vi "Autonomous Independent.vi"   [LabVIEW 2017]
doc: "This VI is called when autonomous begins, and will automatically be terminated when autonomous ends. You can carry out timed or sensor driven robot movement independently without needing to return to the caller."
uses:
  <vilib>/Rock Robotics/WPI/Utilities/WPI_GetSetVariantRefNum.vi
  <vilib>/Rock Robotics/Network Tables/NT Read String.vi
  <vilib>/Rock Robotics/Network Tables/NT Write Numeric Array.vi
  <vilib>/Rock Robotics/WPI/RobotDrive/WPI_RobotDriveArcadeDrive_Standard(NoSaturation).vi
panel:
  # "Be sure to right-click and choose Data Operations>>Make Current Value default if you want to save the array values with the VI"
types:
  T1 = typedef "WPI_JoystickDevRef.ctl" = cluster{"Device":T2}
  T2 = typedef "WPI_JoystickDeviceEnum.ctl" = enum16{"USB 0", "USB 1", "USB 2", "USB 3", "USB 4", "USB 5"}
  T3 = typedef "WPI_RobotDriveDevRef.ctl" = cluster{"DevStatus":errorcluster, "Motors[]":T4[], "Square Inputs":bool, "Max Output":dbl}
  T4 = typedef "WPI_MotorControlDeviceRef.ctl" = cluster{"DeviceStatus":errorcluster, "Type":T5, "PWM":cluster{"PWM Channel":T6, "DeadBand":T7}, "CAN":cluster{"Device Number":u8, "SetOutput VI Ref":variant, "GetOutput VI Ref":variant, "Enable VI Ref":variant, "Disable VI Ref":variant, "Data":variant}, "Invert":bool, "DIO PWM":cluster{"PWM \"Enable\" Channel":T6, "DIOChannel":T8, "PWM Rate":dbl}}
  T5 = typedef "WPI_MotorControlType.ctl" = enum16{"PWM", "CAN", "DIO PWM"}
  T6 = typedef "FPGA_DIOPWMChannel.ctl" = enum8{"PWM 0", "PWM 1", "PWM 2", "PWM 3", "PWM 4", "PWM 5", "PWM 6", "PWM 7", "PWM 8", "PWM 9", "PWM MXP 0", "PWM MXP 1", "PWM MXP 2", "PWM MXP 3", "PWM MXP 4", "PWM MXP 5", "PWM MXP 6", "PWM MXP 7", "PWM MXP 8", "PWM MXP 9", "Invalid"}
  T7 = typedef "WPI_PWMDeadband.ctl" = cluster{"Name":string, "maxPositivePwm":i32, "minPositivePwm":i32, "centerPwm":i32, "maxNegativePwm":i32, "minNegativePwm":i32, "angularRange":u16}
  T8 = typedef "FPGA_DIOChannel.ctl" = enum8{"DIO 0", "DIO 1", "DIO 2", "DIO 3", "DIO 4", "DIO 5", "DIO 6", "DIO 7", "DIO 8", "DIO 9", "DIO MXP 0", "DIO MXP 1", "DIO MXP 2", "DIO MXP 3", "DIO MXP 4", "DIO MXP 5", "DIO MXP 6", "DIO MXP 7", "DIO MXP 8", "DIO MXP 9", "DIO MXP 10", "DIO MXP 11", "DIO MXP 12", "DIO MXP 13", "DIO MXP 14", "DIO MXP 15", "SPI Port CS1", "SPI Port CS2", "SPI Port CS3", "SPI Port MISO", "SPI Port MOSI", "Invalid"}
  T9 = typedef "WPI_SwitchDevRef.ctl" = cluster{"DevStatus":errorcluster, "DIO Channel":T8, "CntIndex":T10, "Normally Closed":bool}
  T10 = typedef "FPGA_CounterCtrSystemIndex.ctl" = enum8{"Ctr 0", "Ctr 1", "Ctr 2", "Ctr 3", "Ctr 4", "Ctr 5", "Ctr 6", "Ctr 7", "Invalid"}
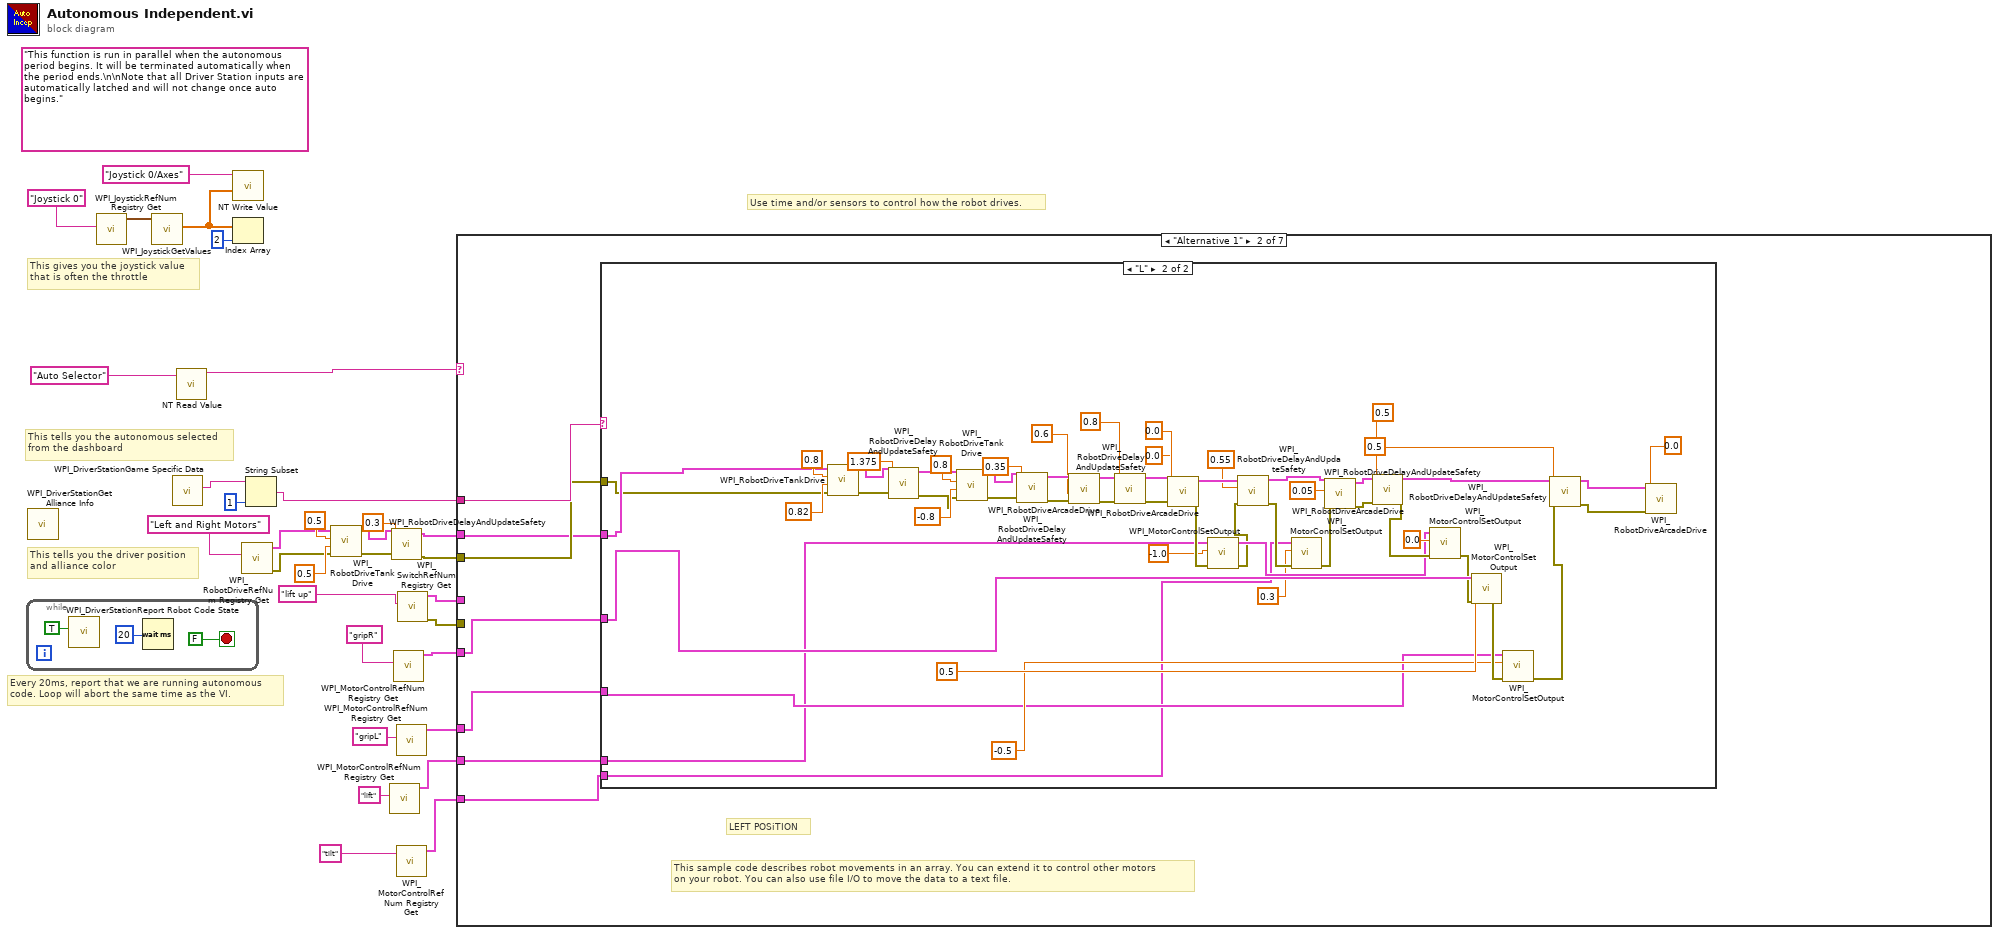
[diagram p0: block diagram]
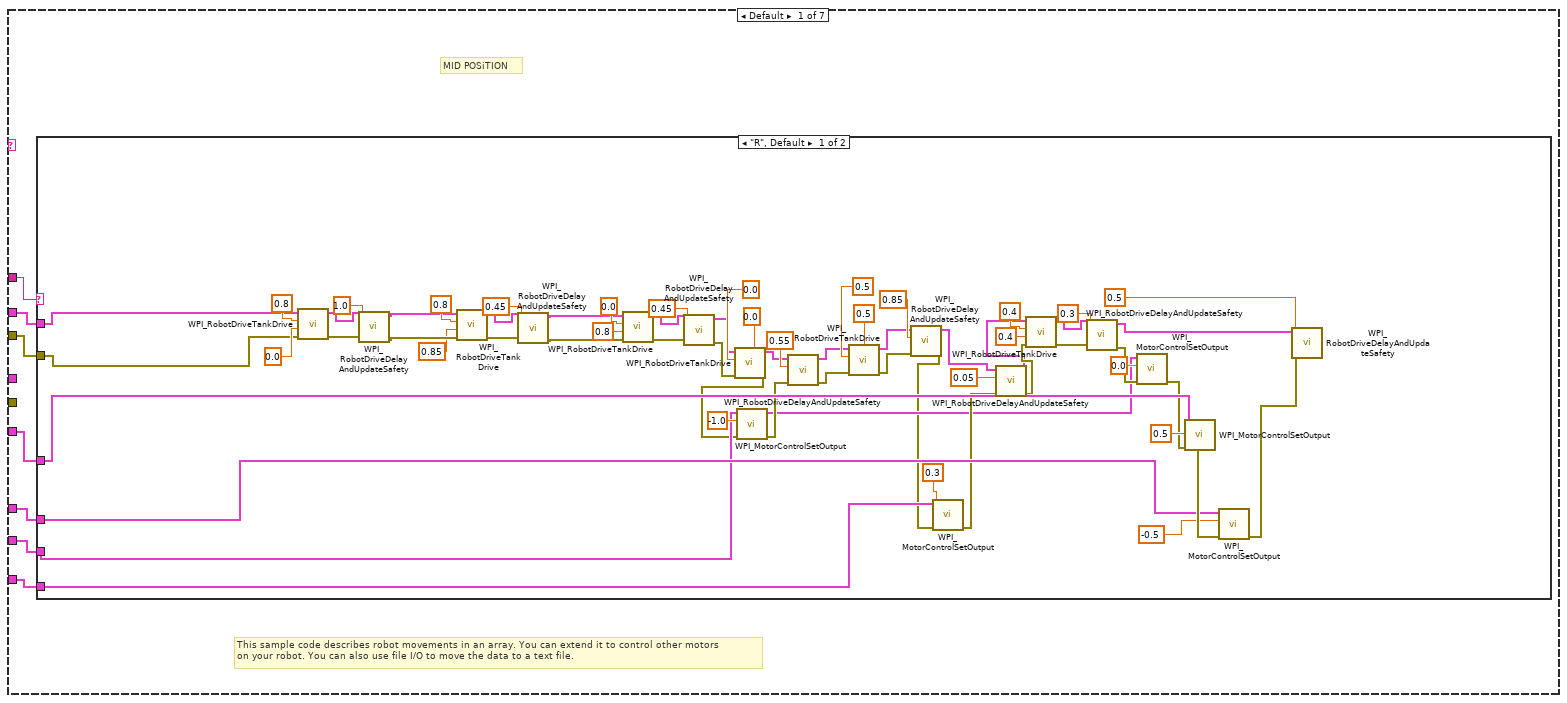
[diagram p2: hidden frame]
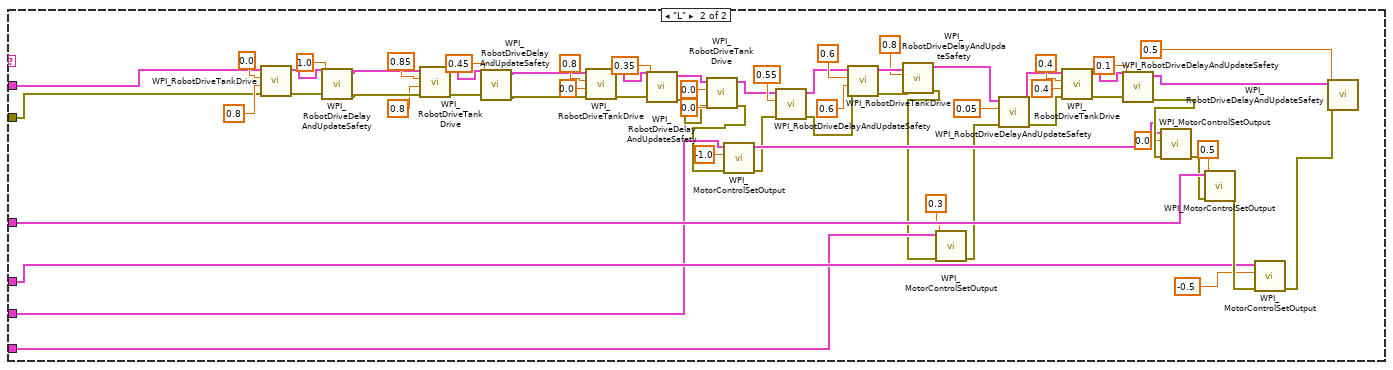
[diagram p3: hidden frame]
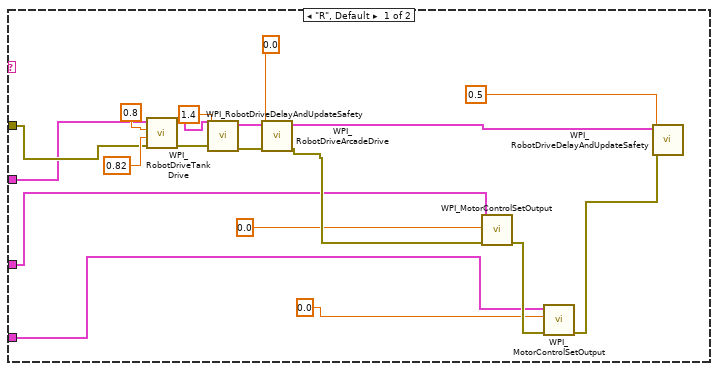
[diagram p4: hidden frame]
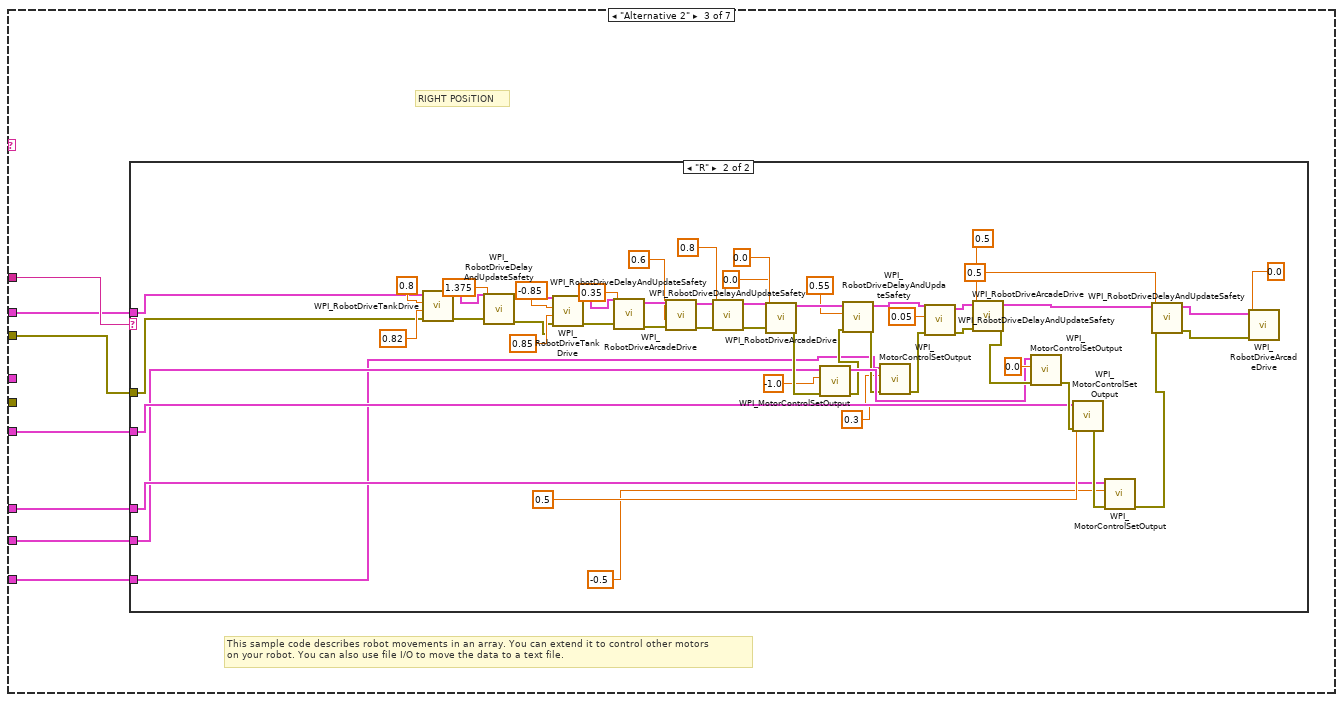
[diagram p5: hidden frame]
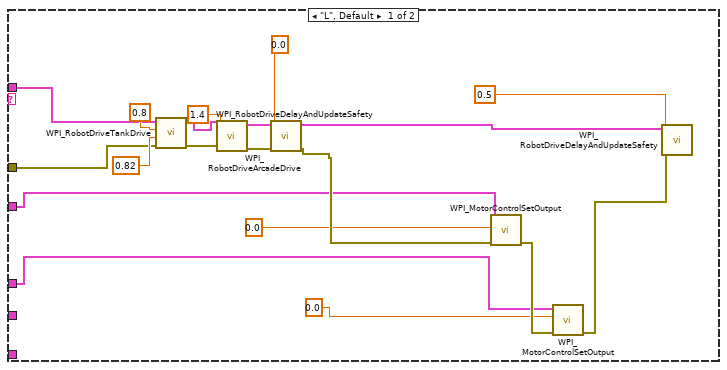
[diagram p6: hidden frame]
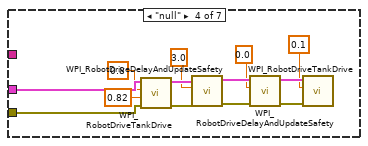
[diagram p7: hidden frame]
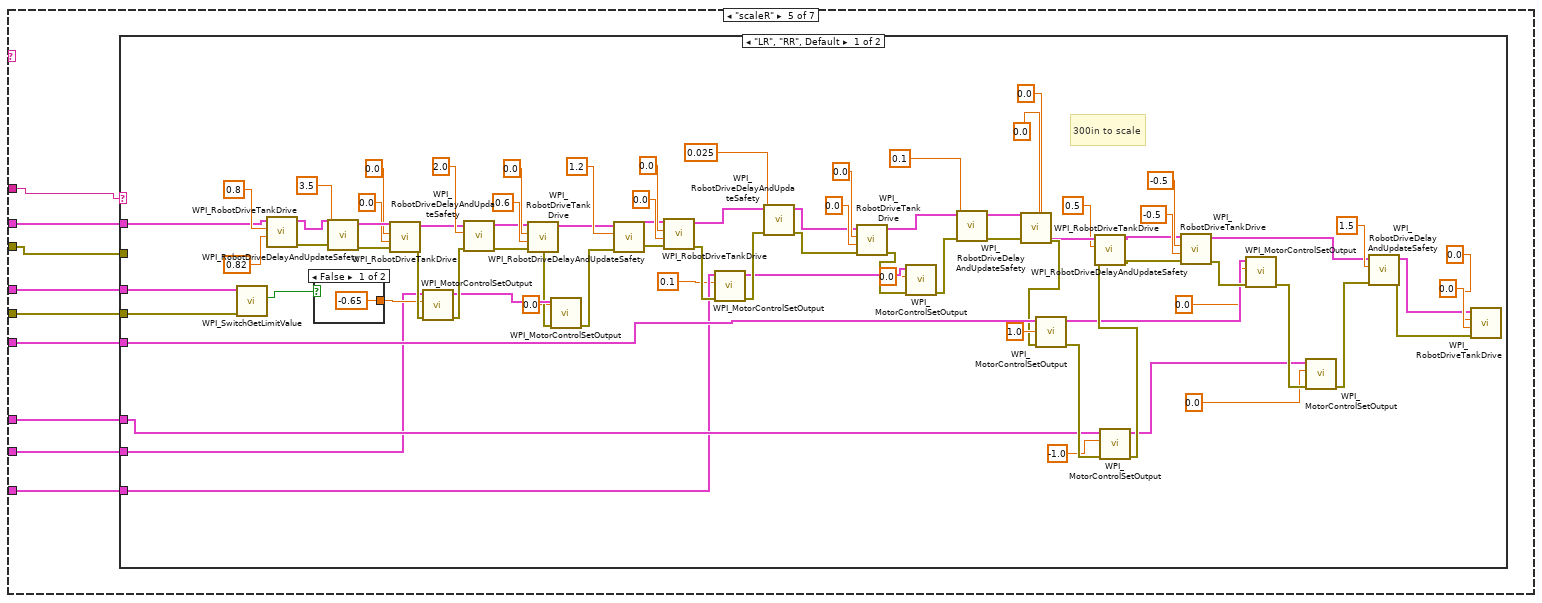
[diagram p8: hidden frame]
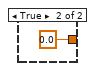
[diagram p9: hidden frame]
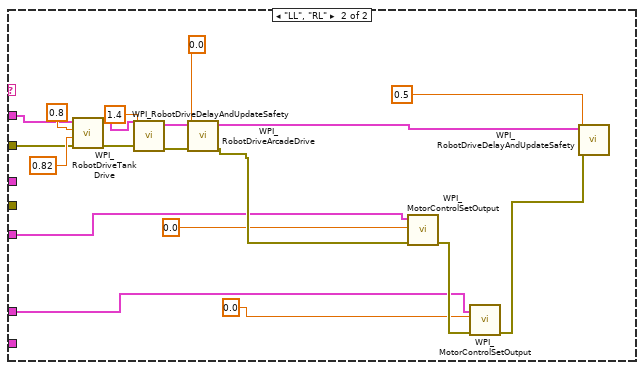
[diagram p10: hidden frame]
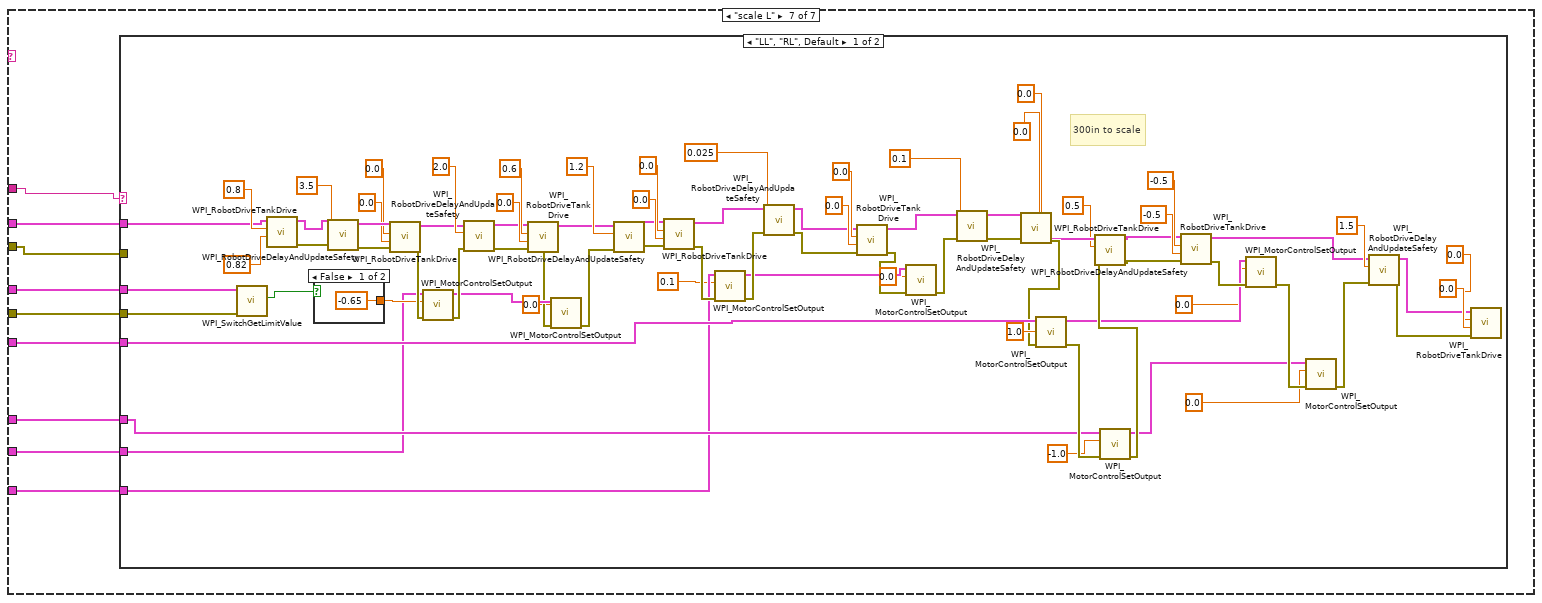
[diagram p12: hidden frame]
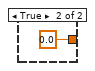
[diagram p13: hidden frame]
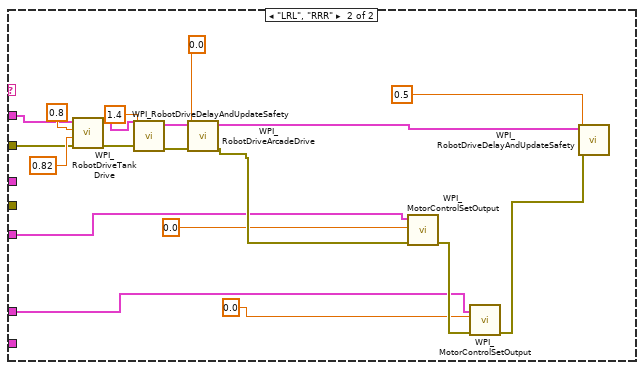
[diagram p14: hidden frame]
diagram:
  (unwired) "This function is run in parallel when the autonomous period begins. It will be terminated automatically when the period ends.\n\nNote that all Driver Station inputs are automatically latched and will not change once auto begins."
  # "This tells you the autonomous selected\nfrom the dashboard"
  # "Every 20ms, report that we are running autonomous\ncode. Loop will abort the same time as the VI."
  # "This gives you the joystick value\nthat is often the throttle"
  # "Use time and/or sensors to control how the robot drives."
  # "This tells you the driver position\nand alliance color"
  n1 = while {
    stop <- FALSE stop-if-true
    n2 = call <vilib>:"WPI_DriverStationReport Robot Code State.vi"("Autonomous"=TRUE) -> ()  [unwired: 10 in, 1 out]
    n3 = Wait (ms)(milliseconds to wait=u32 20) -> ()  [unwired: 1 out]
  }
  n4 = call <vilib>:"WPI_DriverStationGet Alliance Info.vi"() -> ()  [unwired: 12 out]
  n5 = call <vilib>:"WPI_JoystickRefNum Registry Get.vi"("refnum name"="Joystick 0") -> ("JoystickDevRef"=w30:T1)  [unwired: 1 in, 9 out]
  n6 = call <vilib>:"WPI_JoystickGetValues.vi"("JoystickDevRef"=w30) -> ("Axes"=w26:dbl[])  [unwired: 6 in, 4 out]
  n7 = call <vilib>:"WPI_DriverStationGame Specific Data.vi"() -> ("Game Specific Data"=w24:string)  [unwired: 11 in]
  n8 = call-poly <vilib>:"NT Read Value.vi"("Name"="Auto Selector") -> ("String"=w27:string)  [unwired: 9 in, 1 out]
  n9 = call-poly <vilib>:"NT Write Value.vi"("Numeric Array"=w26, "Name"="Joystick 0/Axes") -> ()  [unwired: 9 in, 1 out]
  n10 = Index Array(array=w26, index=2) -> ()  [unwired: 1 out]
  n11 = call <vilib>:"WPI_RobotDriveRefNum Registry Get.vi"("refnum name"="Left and Right Motors") -> ("error out"=w6:errorcluster, "RobotDriveDevRef"=w5:T3)  [unwired: 1 in, 8 out]
  n12 = String Subset(string=w24, length (rest)=1 ("length (rest)")) -> (substring=w22:string)  [unwired: 1 in]
  n13 = call <vilib>:"WPI_RobotDriveTankDrive.vi"("error in (no error)"=w6, "Right axis value"=0.5 ("Y axis value"), "Left axis value"=0.5 ("X axis value"), "RobotDriveDevRef"=w5) -> ("error out"=w10:errorcluster, "RobotDriveDevRef"=w9:T3)  [unwired: 5 in, 1 out]
  n14 = call <vilib>:"WPI_MotorControlRefNum Registry Get.vi"("refnum name"="lift") -> ("MotorControlDevRef"=w12:T4)  [unwired: 9 in, 1 out]
  n15 = call <vilib>:"WPI_RobotDriveDelayAndUpdateSafety.vi"("error in (no error)"=w10, "Delay (s)"=0.3, "RobotDriveDevRef"=w9) -> ("error out"=w3:errorcluster, "RobotDriveDevRef 2"=w4:T3)  [unwired: 7 in]
  n16 = call <vilib>:"WPI_MotorControlRefNum Registry Get.vi"("refnum name"="gripR") -> ("MotorControlDevRef"=w19:T4)  [unwired: 9 in, 1 out]
  n17 = call <vilib>:"WPI_MotorControlRefNum Registry Get.vi"("refnum name"="gripL") -> ("MotorControlDevRef"=w17:T4)  [unwired: 9 in, 1 out]
  n18 = call <vilib>:"WPI_MotorControlRefNum Registry Get.vi"("refnum name"="tilt") -> ("MotorControlDevRef"=w2:T4)  [unwired: 9 in, 1 out]
  n19 = call <vilib>:"WPI_SwitchRefNum Registry Get.vi"("refnum name"="lift up") -> ("error out"=w14:errorcluster, "SwitchDevRef"=w13:T9)  [unwired: 9 in]
  n20 = case shown="\"Alternative 1\"" w27 {
    tunnel: w22 -> [w41 w174 w254 _ w349 _ w458]
    tunnel: w3 -> [w40 w173 w253 w337 w342 _ w451]
    tunnel: w19 -> [w39 w172 w252 _ w346 _ w455]
    tunnel: w17 -> [w38 w171 w251 _ w347 _ w456]
    tunnel: w4 -> [w37 w170 w250 w338 w348 _ w457]
    tunnel: w14 -> [_ _ _ _ w345 _ w454]
    tunnel: w13 -> [_ _ _ _ w344 _ w453]
    tunnel: w12 -> [w36 w169 w249 _ w343 _ w452]
    tunnel: w2 -> [w35 w168 w248 _ w341 _ w450]
    frame Default {
      # "MID POSiTION"
      # "This sample code describes robot movements in an array. You can extend it to control other motors\non your robot. You can also use file I/O to move the data to a text file."
      n21 = case shown="\"R\", Default" w41 {
        tunnel: w40 -> [w94 w137]
        tunnel: w39 -> [w93 w136]
        tunnel: w38 -> [w92 w135]
        tunnel: w37 -> [w71 w134]
        tunnel: w36 -> [w61 w129]
        tunnel: w35 -> [w60 w124]
        frame "R", Default {
          n22 = call <vilib>:"WPI_RobotDriveTankDrive.vi"("error in (no error)"=w94, "Right axis value"=0.0 ("Y axis value"), "Left axis value"=0.8 ("X axis value"), "RobotDriveDevRef"=w71) -> ("error out"=w100:errorcluster, "RobotDriveDevRef"=w99:T3)  [unwired: 5 in, 1 out]
          n23 = call <vilib>:"WPI_RobotDriveDelayAndUpdateSafety.vi"("error in (no error)"=w100, "Delay (s)"=1.0, "RobotDriveDevRef"=w99) -> ("error out"=w86:errorcluster, "RobotDriveDevRef 2"=w87:T3)  [unwired: 7 in]
          n24 = call <vilib>:"WPI_RobotDriveTankDrive.vi"("error in (no error)"=w86, "Right axis value"=0.85, "Left axis value"=0.8 ("X axis value"), "RobotDriveDevRef"=w87) -> ("error out"=w90:errorcluster, "RobotDriveDevRef"=w89:T3)  [unwired: 5 in, 1 out]
          n25 = call <vilib>:"WPI_RobotDriveDelayAndUpdateSafety.vi"("error in (no error)"=w90, "Delay (s)"=0.45, "RobotDriveDevRef"=w89) -> ("error out"=w79:errorcluster, "RobotDriveDevRef 2"=w80:T3)  [unwired: 7 in]
          n26 = call <vilib>:"WPI_RobotDriveTankDrive.vi"("error in (no error)"=w79, "Right axis value"=0.8, "Left axis value"=0.0 ("X axis value"), "RobotDriveDevRef"=w80) -> ("error out"=w83:errorcluster, "RobotDriveDevRef"=w82:T3)  [unwired: 5 in, 1 out]
          n27 = call <vilib>:"WPI_RobotDriveDelayAndUpdateSafety.vi"("error in (no error)"=w83, "Delay (s)"=0.45, "RobotDriveDevRef"=w82) -> ("error out"=w48:errorcluster, "RobotDriveDevRef 2"=w49:T3)  [unwired: 7 in]
          n28 = call <vilib>:"WPI_RobotDriveTankDrive.vi"("error in (no error)"=w48, "Right axis value"=0.0 ("Y axis value"), "Left axis value"=0.0 ("X axis value"), "RobotDriveDevRef"=w49) -> ("error out"=w47:errorcluster, "RobotDriveDevRef"=w46:T3)  [unwired: 5 in, 1 out]
          n29 = call <vilib>:"WPI_MotorControlSetOutput.vi"("error in (no error)"=w47, "Output"=-1.0, "MotorControlDevRef"=w61) -> ("error out"=w64:errorcluster, "MotorControlDevRef"=w59:T4)  [unwired: 6 in, 1 out]
          n30 = call <vilib>:"WPI_RobotDriveDelayAndUpdateSafety.vi"("error in (no error)"=w64, "Delay (s)"=0.55 ("Output"), "RobotDriveDevRef"=w46) -> ("error out"=w45:errorcluster, "RobotDriveDevRef 2"=w44:T3)  [unwired: 7 in]
          n31 = call <vilib>:"WPI_RobotDriveTankDrive.vi"("error in (no error)"=w45, "Right axis value"=0.5 ("Y axis value"), "Left axis value"=0.5 ("X axis value"), "RobotDriveDevRef"=w44) -> ("error out"=w54:errorcluster, "RobotDriveDevRef"=w55:T3)  [unwired: 5 in, 1 out]
          n32 = call <vilib>:"WPI_RobotDriveDelayAndUpdateSafety.vi"("error in (no error)"=w54, "Delay (s)"=0.85, "RobotDriveDevRef"=w55) -> ("error out"=w42:errorcluster, "RobotDriveDevRef 2"=w43:T3)  [unwired: 7 in]
          n33 = call <vilib>:"WPI_MotorControlSetOutput.vi"("error in (no error)"=w42, "Output"=0.3, "MotorControlDevRef"=w60) -> ("error out"=w63:errorcluster)  [unwired: 6 in, 2 out]
          n34 = call <vilib>:"WPI_RobotDriveDelayAndUpdateSafety.vi"("error in (no error)"=w63, "Delay (s)"=0.05, "RobotDriveDevRef"=w43) -> ("error out"=w62:errorcluster, "RobotDriveDevRef 2"=w58:T3)  [unwired: 7 in]
          n35 = call <vilib>:"WPI_RobotDriveTankDrive.vi"("error in (no error)"=w62, "Right axis value"=0.4, "Left axis value"=0.4 ("X axis value"), "RobotDriveDevRef"=w58) -> ("error out"=w76:errorcluster, "RobotDriveDevRef"=w75:T3)  [unwired: 5 in, 1 out]
          n36 = call <vilib>:"WPI_RobotDriveDelayAndUpdateSafety.vi"("error in (no error)"=w76, "Delay (s)"=0.3, "RobotDriveDevRef"=w75) -> ("error out"=w70:errorcluster, "RobotDriveDevRef 2"=w72:T3)  [unwired: 7 in]
          n37 = call <vilib>:"WPI_MotorControlSetOutput.vi"("error in (no error)"=w70, "Output"=0.0, "MotorControlDevRef"=w59) -> ("error out"=w68:errorcluster)  [unwired: 6 in, 2 out]
          n38 = call <vilib>:"WPI_MotorControlSetOutput.vi"("error in (no error)"=w68, "Output"=0.5, "MotorControlDevRef"=w93) -> ("error out"=w102:errorcluster)  [unwired: 6 in, 2 out]
          n39 = call <vilib>:"WPI_MotorControlSetOutput.vi"("error in (no error)"=w102, "Output"=-0.5, "MotorControlDevRef"=w92) -> ("error out"=w101:errorcluster)  [unwired: 6 in, 2 out]
          n40 = call <vilib>:"WPI_RobotDriveDelayAndUpdateSafety.vi"("error in (no error)"=w101, "Delay (s)"=0.5, "RobotDriveDevRef"=w72) -> ()  [unwired: 7 in, 2 out]
        }
        frame "L" {
          n41 = call <vilib>:"WPI_RobotDriveTankDrive.vi"("error in (no error)"=w137, "Right axis value"=0.8 ("Y axis value"), "Left axis value"=0.0 ("X axis value"), "RobotDriveDevRef"=w134) -> ("error out"=w163:errorcluster, "RobotDriveDevRef"=w162:T3)  [unwired: 5 in, 1 out]
          n42 = call <vilib>:"WPI_RobotDriveDelayAndUpdateSafety.vi"("error in (no error)"=w163, "Delay (s)"=1.0, "RobotDriveDevRef"=w162) -> ("error out"=w152:errorcluster, "RobotDriveDevRef 2"=w153:T3)  [unwired: 7 in]
          n43 = call <vilib>:"WPI_RobotDriveTankDrive.vi"("error in (no error)"=w152, "Right axis value"=0.8, "Left axis value"=0.85 ("X axis value"), "RobotDriveDevRef"=w153) -> ("error out"=w156:errorcluster, "RobotDriveDevRef"=w155:T3)  [unwired: 5 in, 1 out]
          n44 = call <vilib>:"WPI_RobotDriveDelayAndUpdateSafety.vi"("error in (no error)"=w156, "Delay (s)"=0.45, "RobotDriveDevRef"=w155) -> ("error out"=w145:errorcluster, "RobotDriveDevRef 2"=w146:T3)  [unwired: 7 in]
          n45 = call <vilib>:"WPI_RobotDriveTankDrive.vi"("error in (no error)"=w145, "Right axis value"=0.0, "Left axis value"=0.8 ("X axis value"), "RobotDriveDevRef"=w146) -> ("error out"=w149:errorcluster, "RobotDriveDevRef"=w148:T3)  [unwired: 5 in, 1 out]
          n46 = call <vilib>:"WPI_RobotDriveDelayAndUpdateSafety.vi"("error in (no error)"=w149, "Delay (s)"=0.35, "RobotDriveDevRef"=w148) -> ("error out"=w111:errorcluster, "RobotDriveDevRef 2"=w112:T3)  [unwired: 7 in]
          n47 = call <vilib>:"WPI_RobotDriveTankDrive.vi"("error in (no error)"=w111, "Right axis value"=0.0, "Left axis value"=0.0, "RobotDriveDevRef"=w112) -> ("error out"=w109:errorcluster, "RobotDriveDevRef"=w110:T3)  [unwired: 5 in, 1 out]
          n48 = call <vilib>:"WPI_MotorControlSetOutput.vi"("error in (no error)"=w109, "Output"=-1.0, "MotorControlDevRef"=w129) -> ("error out"=w122:errorcluster, "MotorControlDevRef"=w126:T4)  [unwired: 6 in, 1 out]
          n49 = call <vilib>:"WPI_RobotDriveDelayAndUpdateSafety.vi"("error in (no error)"=w122, "Delay (s)"=0.55 ("Output"), "RobotDriveDevRef"=w110) -> ("error out"=w106:errorcluster, "RobotDriveDevRef 2"=w108:T3)  [unwired: 7 in]
          n50 = call <vilib>:"WPI_RobotDriveTankDrive.vi"("error in (no error)"=w106, "Right axis value"=0.6 ("X axis value"), "Left axis value"=0.6 ("X axis value"), "RobotDriveDevRef"=w108) -> ("error out"=w118:errorcluster, "RobotDriveDevRef"=w119:T3)  [unwired: 5 in, 1 out]
          n51 = call <vilib>:"WPI_RobotDriveDelayAndUpdateSafety.vi"("error in (no error)"=w118, "Delay (s)"=0.8 ("X axis value"), "RobotDriveDevRef"=w119) -> ("error out"=w105:errorcluster, "RobotDriveDevRef 2"=w107:T3)  [unwired: 7 in]
          n52 = call <vilib>:"WPI_MotorControlSetOutput.vi"("error in (no error)"=w105, "Output"=0.3, "MotorControlDevRef"=w124) -> ("error out"=w121:errorcluster)  [unwired: 6 in, 2 out]
          n53 = call <vilib>:"WPI_RobotDriveDelayAndUpdateSafety.vi"("error in (no error)"=w121, "Delay (s)"=0.05, "RobotDriveDevRef"=w107) -> ("error out"=w130:errorcluster, "RobotDriveDevRef 2"=w131:T3)  [unwired: 7 in]
          n54 = call <vilib>:"WPI_RobotDriveTankDrive.vi"("error in (no error)"=w130, "Right axis value"=0.4, "Left axis value"=0.4 ("X axis value"), "RobotDriveDevRef"=w131) -> ("error out"=w142:errorcluster, "RobotDriveDevRef"=w141:T3)  [unwired: 5 in, 1 out]
          n55 = call <vilib>:"WPI_RobotDriveDelayAndUpdateSafety.vi"("error in (no error)"=w142, "Delay (s)"=0.1, "RobotDriveDevRef"=w141) -> ("error out"=w128:errorcluster, "RobotDriveDevRef 2"=w138:T3)  [unwired: 7 in]
          n56 = call <vilib>:"WPI_MotorControlSetOutput.vi"("error in (no error)"=w128, "Output"=0.0, "MotorControlDevRef"=w126) -> ("error out"=w127:errorcluster)  [unwired: 6 in, 2 out]
          n57 = call <vilib>:"WPI_MotorControlSetOutput.vi"("error in (no error)"=w127, "Output"=0.5, "MotorControlDevRef"=w136) -> ("error out"=w165:errorcluster)  [unwired: 6 in, 2 out]
          n58 = call <vilib>:"WPI_MotorControlSetOutput.vi"("error in (no error)"=w165, "Output"=-0.5, "MotorControlDevRef"=w135) -> ("error out"=w164:errorcluster)  [unwired: 6 in, 2 out]
          n59 = call <vilib>:"WPI_RobotDriveDelayAndUpdateSafety.vi"("error in (no error)"=w164, "Delay (s)"=0.5, "RobotDriveDevRef"=w138) -> ()  [unwired: 7 in, 2 out]
        }
      }
    }
    frame "Alternative 1" {
      # "LEFT POSiTION"
      # "This sample code describes robot movements in an array. You can extend it to control other motors\non your robot. You can also use file I/O to move the data to a text file."
      n60 = case shown="\"L\"" w174 {
        tunnel: w173 -> [w178 w227]
        tunnel: w172 -> [w177 w226]
        tunnel: w171 -> [w176 w225]
        tunnel: w170 -> [w175 w228]
        tunnel: w169 -> [_ w205]
        tunnel: w168 -> [_ w195]
        frame "R", Default {
          n61 = call <vilib>:"WPI_RobotDriveTankDrive.vi"("error in (no error)"=w178, "Right axis value"=0.82 ("Y axis value"), "Left axis value"=0.8 ("X axis value"), "RobotDriveDevRef"=w175) -> ("error out"=w184:errorcluster, "RobotDriveDevRef"=w183:T3)  [unwired: 5 in, 1 out]
          n62 = call <vilib>:"WPI_RobotDriveDelayAndUpdateSafety.vi"("error in (no error)"=w184, "Delay (s)"=1.4, "RobotDriveDevRef"=w183) -> ("error out"=w192:errorcluster, "RobotDriveDevRef 2"=w191:T3)  [unwired: 7 in]
          n63 = call-poly <vilib>:"WPI_RobotDriveArcadeDrive.vi"("error in (no error)"=w192, "Y axis value"=0.0, "RobotDriveDevRef"=w191) -> ("error out"=w186:errorcluster, "RobotDriveDevRef"=w189:T3)  [unwired: 6 in, 1 out]
          n64 = call <vilib>:"WPI_MotorControlSetOutput.vi"("error in (no error)"=w186, "Output"=0.0, "MotorControlDevRef"=w177) -> ("error out"=w187:errorcluster)  [unwired: 6 in, 2 out]
          n65 = call <vilib>:"WPI_MotorControlSetOutput.vi"("error in (no error)"=w187, "Output"=0.0, "MotorControlDevRef"=w176) -> ("error out"=w185:errorcluster)  [unwired: 6 in, 2 out]
          n66 = call <vilib>:"WPI_RobotDriveDelayAndUpdateSafety.vi"("error in (no error)"=w185, "Delay (s)"=0.5, "RobotDriveDevRef"=w189) -> ()  [unwired: 7 in, 2 out]
        }
        frame "L" {
          n67 = call <vilib>:"WPI_RobotDriveTankDrive.vi"("error in (no error)"=w227, "Right axis value"=0.82 ("Y axis value"), "Left axis value"=0.8 ("X axis value"), "RobotDriveDevRef"=w228) -> ("error out"=w241:errorcluster, "RobotDriveDevRef"=w240:T3)  [unwired: 5 in, 1 out]
          n68 = call <vilib>:"WPI_RobotDriveDelayAndUpdateSafety.vi"("error in (no error)"=w241, "Delay (s)"=1.375, "RobotDriveDevRef"=w240) -> ("error out"=w229:errorcluster, "RobotDriveDevRef 2"=w230:T3)  [unwired: 7 in]
          n69 = call <vilib>:"WPI_RobotDriveTankDrive.vi"("error in (no error)"=w229, "Right axis value"=-0.8 ("Y axis value"), "Left axis value"=0.8 ("X axis value"), "RobotDriveDevRef"=w230) -> ("error out"=w234:errorcluster, "RobotDriveDevRef"=w233:T3)  [unwired: 5 in, 1 out]
          n70 = call <vilib>:"WPI_RobotDriveDelayAndUpdateSafety.vi"("error in (no error)"=w234, "Delay (s)"=0.35, "RobotDriveDevRef"=w233) -> ("error out"=w220:errorcluster, "RobotDriveDevRef 2"=w221:T3)  [unwired: 7 in]
          n71 = call-poly <vilib>:"WPI_RobotDriveArcadeDrive.vi"("error in (no error)"=w220, "Y axis value"=0.6, "RobotDriveDevRef"=w221) -> ("error out"=w217:errorcluster, "RobotDriveDevRef"=w218:T3)  [unwired: 6 in, 1 out]
          n72 = call <vilib>:"WPI_RobotDriveDelayAndUpdateSafety.vi"("error in (no error)"=w217, "Delay (s)"=0.8, "RobotDriveDevRef"=w218) -> ("error out"=w215:errorcluster, "RobotDriveDevRef 2"=w214:T3)  [unwired: 7 in]
          n73 = call-poly <vilib>:"WPI_RobotDriveArcadeDrive.vi"("error in (no error)"=w215, "Y axis value"=0.0, "X axis value"=0.0, "RobotDriveDevRef"=w214) -> ("error out"=w206:errorcluster, "RobotDriveDevRef"=w202:T3)  [unwired: 5 in, 1 out]
          n74 = call <vilib>:"WPI_MotorControlSetOutput.vi"("error in (no error)"=w206, "Output"=-1.0 ("Delay (s)"), "MotorControlDevRef"=w205) -> ("error out"=w201:errorcluster, "MotorControlDevRef"=w204:T4)  [unwired: 6 in, 1 out]
          n75 = call <vilib>:"WPI_RobotDriveDelayAndUpdateSafety.vi"("error in (no error)"=w201, "Delay (s)"=0.55, "RobotDriveDevRef"=w202) -> ("error out"=w198:errorcluster, "RobotDriveDevRef 2"=w199:T3)  [unwired: 7 in]
          n76 = call <vilib>:"WPI_MotorControlSetOutput.vi"("error in (no error)"=w198, "Output"=0.3 ("Delay (s)"), "MotorControlDevRef"=w195) -> ("error out"=w197:errorcluster)  [unwired: 6 in, 2 out]
          n77 = call <vilib>:"WPI_RobotDriveDelayAndUpdateSafety.vi"("error in (no error)"=w197, "Delay (s)"=0.05, "RobotDriveDevRef"=w199) -> ("error out"=w194:errorcluster, "RobotDriveDevRef 2"=w213:T3)  [unwired: 7 in]
          n78 = call-poly <vilib>:"WPI_RobotDriveArcadeDrive.vi"("error in (no error)"=w194, "Y axis value"=0.5, "RobotDriveDevRef"=w213) -> ("error out"=w208:errorcluster, "RobotDriveDevRef"=w245:T3)  [unwired: 6 in, 1 out]
          n79 = call <vilib>:"WPI_MotorControlSetOutput.vi"("error in (no error)"=w208, "Output"=0.0, "MotorControlDevRef"=w204) -> ("error out"=w207:errorcluster)  [unwired: 6 in, 2 out]
          n80 = call <vilib>:"WPI_MotorControlSetOutput.vi"("error in (no error)"=w207, "Output"=0.5, "MotorControlDevRef"=w226) -> ("error out"=w243:errorcluster)  [unwired: 6 in, 2 out]
          n81 = call <vilib>:"WPI_MotorControlSetOutput.vi"("error in (no error)"=w243, "Output"=-0.5, "MotorControlDevRef"=w225) -> ("error out"=w242:errorcluster)  [unwired: 6 in, 2 out]
          n82 = call <vilib>:"WPI_RobotDriveDelayAndUpdateSafety.vi"("error in (no error)"=w242, "Delay (s)"=0.5, "RobotDriveDevRef"=w245) -> ("error out"=w222:errorcluster, "RobotDriveDevRef 2"=w223:T3)  [unwired: 7 in]
          n83 = call-poly <vilib>:"WPI_RobotDriveArcadeDrive.vi"("error in (no error)"=w222, "Y axis value"=0.0, "RobotDriveDevRef"=w223) -> ()  [unwired: 6 in, 3 out]
        }
      }
    }
    frame "Alternative 2" {
      # "RIGHT POSiTION"
      # "This sample code describes robot movements in an array. You can extend it to control other motors\non your robot. You can also use file I/O to move the data to a text file."
      n84 = case shown="\"R\"" w254 {
        tunnel: w253 -> [w256 w289]
        tunnel: w252 -> [w257 w288]
        tunnel: w251 -> [w258 w287]
        tunnel: w250 -> [w255 w290]
        tunnel: w249 -> [_ w285]
        tunnel: w248 -> [_ w274]
        frame "L", Default {
          n85 = call <vilib>:"WPI_RobotDriveTankDrive.vi"("error in (no error)"=w256, "Right axis value"=0.82 ("Y axis value"), "Left axis value"=0.8 ("X axis value"), "RobotDriveDevRef"=w255) -> ("error out"=w264:errorcluster, "RobotDriveDevRef"=w263:T3)  [unwired: 5 in, 1 out]
          n86 = call <vilib>:"WPI_RobotDriveDelayAndUpdateSafety.vi"("error in (no error)"=w264, "Delay (s)"=1.4, "RobotDriveDevRef"=w263) -> ("error out"=w272:errorcluster, "RobotDriveDevRef 2"=w271:T3)  [unwired: 7 in]
          n87 = call-poly <vilib>:"WPI_RobotDriveArcadeDrive.vi"("error in (no error)"=w272, "Y axis value"=0.0, "RobotDriveDevRef"=w271) -> ("error out"=w266:errorcluster, "RobotDriveDevRef"=w269:T3)  [unwired: 6 in, 1 out]
          n88 = call <vilib>:"WPI_MotorControlSetOutput.vi"("error in (no error)"=w266, "Output"=0.0, "MotorControlDevRef"=w257) -> ("error out"=w267:errorcluster)  [unwired: 6 in, 2 out]
          n89 = call <vilib>:"WPI_MotorControlSetOutput.vi"("error in (no error)"=w267, "Output"=0.0, "MotorControlDevRef"=w258) -> ("error out"=w265:errorcluster)  [unwired: 6 in, 2 out]
          n90 = call <vilib>:"WPI_RobotDriveDelayAndUpdateSafety.vi"("error in (no error)"=w265, "Delay (s)"=0.5, "RobotDriveDevRef"=w269) -> ()  [unwired: 7 in, 2 out]
        }
        frame "R" {
          n91 = call <vilib>:"WPI_RobotDriveTankDrive.vi"("error in (no error)"=w289, "Right axis value"=0.82 ("Y axis value"), "Left axis value"=0.8 ("X axis value"), "RobotDriveDevRef"=w290) -> ("error out"=w321:errorcluster, "RobotDriveDevRef"=w320:T3)  [unwired: 5 in, 1 out]
          n92 = call <vilib>:"WPI_RobotDriveDelayAndUpdateSafety.vi"("error in (no error)"=w321, "Delay (s)"=1.375, "RobotDriveDevRef"=w320) -> ("error out"=w309:errorcluster, "RobotDriveDevRef 2"=w310:T3)  [unwired: 7 in]
          n93 = call <vilib>:"WPI_RobotDriveTankDrive.vi"("error in (no error)"=w309, "Right axis value"=0.85 ("Y axis value"), "Left axis value"=-0.85 ("X axis value"), "RobotDriveDevRef"=w310) -> ("error out"=w314:errorcluster, "RobotDriveDevRef"=w313:T3)  [unwired: 5 in, 1 out]
          n94 = call <vilib>:"WPI_RobotDriveDelayAndUpdateSafety.vi"("error in (no error)"=w314, "Delay (s)"=0.35, "RobotDriveDevRef"=w313) -> ("error out"=w304:errorcluster, "RobotDriveDevRef 2"=w305:T3)  [unwired: 7 in]
          n95 = call-poly <vilib>:"WPI_RobotDriveArcadeDrive.vi"("error in (no error)"=w304, "Y axis value"=0.6, "RobotDriveDevRef"=w305) -> ("error out"=w301:errorcluster, "RobotDriveDevRef"=w302:T3)  [unwired: 6 in, 1 out]
          n96 = call <vilib>:"WPI_RobotDriveDelayAndUpdateSafety.vi"("error in (no error)"=w301, "Delay (s)"=0.8, "RobotDriveDevRef"=w302) -> ("error out"=w299:errorcluster, "RobotDriveDevRef 2"=w298:T3)  [unwired: 7 in]
          n97 = call-poly <vilib>:"WPI_RobotDriveArcadeDrive.vi"("error in (no error)"=w299, "Y axis value"=0.0, "X axis value"=0.0, "RobotDriveDevRef"=w298) -> ("error out"=w286:errorcluster, "RobotDriveDevRef"=w280:T3)  [unwired: 5 in, 1 out]
          n98 = call <vilib>:"WPI_MotorControlSetOutput.vi"("error in (no error)"=w286, "Output"=-1.0 ("Delay (s)"), "MotorControlDevRef"=w285) -> ("error out"=w283:errorcluster, "MotorControlDevRef"=w284:T4)  [unwired: 6 in, 1 out]
          n99 = call <vilib>:"WPI_RobotDriveDelayAndUpdateSafety.vi"("error in (no error)"=w283, "Delay (s)"=0.55, "RobotDriveDevRef"=w280) -> ("error out"=w282:errorcluster, "RobotDriveDevRef 2"=w279:T3)  [unwired: 7 in]
          n100 = call <vilib>:"WPI_MotorControlSetOutput.vi"("error in (no error)"=w282, "Output"=0.3 ("Delay (s)"), "MotorControlDevRef"=w274) -> ("error out"=w281:errorcluster)  [unwired: 6 in, 2 out]
          n101 = call <vilib>:"WPI_RobotDriveDelayAndUpdateSafety.vi"("error in (no error)"=w281, "Delay (s)"=0.05, "RobotDriveDevRef"=w279) -> ("error out"=w275:errorcluster, "RobotDriveDevRef 2"=w297:T3)  [unwired: 7 in]
          n102 = call-poly <vilib>:"WPI_RobotDriveArcadeDrive.vi"("error in (no error)"=w275, "Y axis value"=0.5, "RobotDriveDevRef"=w297) -> ("error out"=w292:errorcluster, "RobotDriveDevRef"=w325:T3)  [unwired: 6 in, 1 out]
          n103 = call <vilib>:"WPI_MotorControlSetOutput.vi"("error in (no error)"=w292, "Output"=0.0, "MotorControlDevRef"=w284) -> ("error out"=w291:errorcluster)  [unwired: 6 in, 2 out]
          n104 = call <vilib>:"WPI_MotorControlSetOutput.vi"("error in (no error)"=w291, "Output"=0.5, "MotorControlDevRef"=w288) -> ("error out"=w323:errorcluster)  [unwired: 6 in, 2 out]
          n105 = call <vilib>:"WPI_MotorControlSetOutput.vi"("error in (no error)"=w323, "Output"=-0.5, "MotorControlDevRef"=w287) -> ("error out"=w322:errorcluster)  [unwired: 6 in, 2 out]
          n106 = call <vilib>:"WPI_RobotDriveDelayAndUpdateSafety.vi"("error in (no error)"=w322, "Delay (s)"=0.5, "RobotDriveDevRef"=w325) -> ("error out"=w306:errorcluster, "RobotDriveDevRef 2"=w307:T3)  [unwired: 7 in]
          n107 = call-poly <vilib>:"WPI_RobotDriveArcadeDrive.vi"("error in (no error)"=w306, "Y axis value"=0.0, "RobotDriveDevRef"=w307) -> ()  [unwired: 6 in, 3 out]
        }
      }
    }
    frame "null" {
      n108 = call <vilib>:"WPI_RobotDriveTankDrive.vi"("error in (no error)"=w337, "Right axis value"=0.82, "Left axis value"=0.8 ("Output"), "RobotDriveDevRef"=w338) -> ("error out"=w340:errorcluster, "RobotDriveDevRef"=w339:T3)  [unwired: 5 in, 1 out]
      n109 = call <vilib>:"WPI_RobotDriveDelayAndUpdateSafety.vi"("error in (no error)"=w340, "Delay (s)"=3.0 ("Output"), "RobotDriveDevRef"=w339) -> ("error out"=w336:errorcluster, "RobotDriveDevRef 2"=w335:T3)  [unwired: 7 in]
      n110 = call <vilib>:"WPI_RobotDriveTankDrive.vi"("error in (no error)"=w336, "Left axis value"=0.0 ("Output"), "RobotDriveDevRef"=w335) -> ("error out"=w334:errorcluster, "RobotDriveDevRef"=w333:T3)  [unwired: 6 in, 1 out]
      n111 = call <vilib>:"WPI_RobotDriveDelayAndUpdateSafety.vi"("error in (no error)"=w334, "Delay (s)"=0.1 ("Output"), "RobotDriveDevRef"=w333) -> ()  [unwired: 7 in, 2 out]
    }
    frame "scaleR" {
      n112 = case shown="\"LR\", \"RR\", Default" w349 {
        tunnel: w348 -> [w419 w433]
        tunnel: w347 -> [w399 w431]
        tunnel: w346 -> [w400 w432]
        tunnel: w345 -> [w396 _]
        tunnel: w344 -> [w395 _]
        tunnel: w343 -> [w394 _]
        tunnel: w342 -> [_ w434]
        tunnel: w341 -> [w363 _]
        frame "LR", "RR", Default {
          # "300in to scale"
          n113 = call <vilib>:"WPI_SwitchGetLimitValue.vi"("error in (no error)"=w396, "SwitchDevRef"=w395) -> ("Switch Pressed"=w397:bool)  [unwired: 7 in, 2 out]
          n114 = call <vilib>:"WPI_RobotDriveTankDrive.vi"("Right axis value"=0.82 ("Y axis value"), "Left axis value"=0.8 ("X axis value"), "RobotDriveDevRef"=w419) -> ("error out"=w425:errorcluster, "RobotDriveDevRef"=w424:T3)  [unwired: 6 in, 1 out]
          n115 = case shown="False" w397 {
            tunnel: [-0.65 ("Output") 0.0 ("Output")] -> w398
            frame False {
            }
            frame True {
            }
          }
          n116 = call <vilib>:"WPI_RobotDriveDelayAndUpdateSafety.vi"("error in (no error)"=w425, "Delay (s)"=3.5, "RobotDriveDevRef"=w424) -> ("error out"=w417:errorcluster, "RobotDriveDevRef 2"=w418:T3)  [unwired: 7 in]
          n117 = call <vilib>:"WPI_RobotDriveTankDrive.vi"("error in (no error)"=w417, "Right axis value"=0.0, "Left axis value"=0.0, "RobotDriveDevRef"=w418) -> ("error out"=w414:errorcluster, "RobotDriveDevRef"=w412:T3)  [unwired: 5 in, 1 out]
          n118 = call <vilib>:"WPI_MotorControlSetOutput.vi"("error in (no error)"=w414, "Output"=w398, "MotorControlDevRef"=w394) -> ("error out"=w411:errorcluster, "MotorControlDevRef"=w393:T4)  [unwired: 6 in, 1 out]
          n119 = call <vilib>:"WPI_RobotDriveDelayAndUpdateSafety.vi"("error in (no error)"=w411, "Delay (s)"=2.0, "RobotDriveDevRef"=w412) -> ("error out"=w405:errorcluster, "RobotDriveDevRef 2"=w406:T3)  [unwired: 7 in]
          n120 = call <vilib>:"WPI_RobotDriveTankDrive.vi"("error in (no error)"=w405, "Right axis value"=0.6, "Left axis value"=0.0, "RobotDriveDevRef"=w406) -> ("error out"=w392:errorcluster, "RobotDriveDevRef"=w407:T3)  [unwired: 5 in, 1 out]
          n121 = call <vilib>:"WPI_MotorControlSetOutput.vi"("error in (no error)"=w392, "Output"=0.0, "MotorControlDevRef"=w393) -> ("error out"=w366:errorcluster)  [unwired: 6 in, 2 out]
          n122 = call <vilib>:"WPI_RobotDriveDelayAndUpdateSafety.vi"("error in (no error)"=w366, "Delay (s)"=1.2, "RobotDriveDevRef"=w407) -> ("error out"=w401:errorcluster, "RobotDriveDevRef 2"=w402:T3)  [unwired: 7 in]
          n123 = call <vilib>:"WPI_RobotDriveTankDrive.vi"("error in (no error)"=w401, "Right axis value"=0.0, "Left axis value"=0.0, "RobotDriveDevRef"=w402) -> ("error out"=w365:errorcluster, "RobotDriveDevRef"=w377:T3)  [unwired: 5 in, 1 out]
          n124 = call <vilib>:"WPI_MotorControlSetOutput.vi"("error in (no error)"=w365, "Output"=0.1, "MotorControlDevRef"=w363) -> ("error out"=w364:errorcluster, "MotorControlDevRef"=w355:T4)  [unwired: 6 in, 1 out]
          n125 = call <vilib>:"WPI_RobotDriveDelayAndUpdateSafety.vi"("error in (no error)"=w364, "Delay (s)"=0.025, "RobotDriveDevRef"=w377) -> ("error out"=w356:errorcluster, "RobotDriveDevRef 2"=w357:T3)  [unwired: 7 in]
          n126 = call <vilib>:"WPI_RobotDriveTankDrive.vi"("error in (no error)"=w356, "Right axis value"=0.0, "Left axis value"=0.0, "RobotDriveDevRef"=w357) -> ("error out"=w353:errorcluster, "RobotDriveDevRef"=w360:T3)  [unwired: 5 in, 1 out]
          n127 = call <vilib>:"WPI_MotorControlSetOutput.vi"("error in (no error)"=w353, "Output"=0.0, "MotorControlDevRef"=w355) -> ("error out"=w352:errorcluster)  [unwired: 6 in, 2 out]
          n128 = call <vilib>:"WPI_RobotDriveDelayAndUpdateSafety.vi"("error in (no error)"=w352, "Delay (s)"=0.1, "RobotDriveDevRef"=w360) -> ("error out"=w350:errorcluster, "RobotDriveDevRef 2"=w351:T3)  [unwired: 7 in]
          n129 = call <vilib>:"WPI_RobotDriveTankDrive.vi"("error in (no error)"=w350, "Right axis value"=0.0, "Left axis value"=0.0, "RobotDriveDevRef"=w351) -> ("error out"=w376:errorcluster, "RobotDriveDevRef"=w375:T3)  [unwired: 5 in, 1 out]
          n130 = call <vilib>:"WPI_MotorControlSetOutput.vi"("error in (no error)"=w376, "Output"=1.0, "MotorControlDevRef"=w400) -> ("error out"=w427:errorcluster, "MotorControlDevRef"=w384:T4)  [unwired: 6 in, 1 out]
          n131 = call <vilib>:"WPI_MotorControlSetOutput.vi"("error in (no error)"=w427, "Output"=-1.0, "MotorControlDevRef"=w399) -> ("error out"=w426:errorcluster, "MotorControlDevRef"=w383:T4)  [unwired: 6 in, 1 out]
          n132 = call <vilib>:"WPI_RobotDriveDelayAndUpdateSafety.vi"("error in (no error)"=w426, "Delay (s)"=0.5, "RobotDriveDevRef"=w375) -> ("error out"=w387:errorcluster, "RobotDriveDevRef 2"=w388:T3)  [unwired: 7 in]
          n133 = call <vilib>:"WPI_RobotDriveTankDrive.vi"("error in (no error)"=w387, "Right axis value"=-0.5, "Left axis value"=-0.5, "RobotDriveDevRef"=w388) -> ("error out"=w385:errorcluster, "RobotDriveDevRef"=w372:T3)  [unwired: 5 in, 1 out]
          n134 = call <vilib>:"WPI_MotorControlSetOutput.vi"("error in (no error)"=w385, "Output"=0.0, "MotorControlDevRef"=w384) -> ("error out"=w386:errorcluster)  [unwired: 6 in, 2 out]
          n135 = call <vilib>:"WPI_MotorControlSetOutput.vi"("error in (no error)"=w386, "Output"=0.0, "MotorControlDevRef"=w383) -> ("error out"=w371:errorcluster)  [unwired: 6 in, 2 out]
          n136 = call <vilib>:"WPI_RobotDriveDelayAndUpdateSafety.vi"("error in (no error)"=w371, "Delay (s)"=1.5, "RobotDriveDevRef"=w372) -> ("error out"=w367:errorcluster, "RobotDriveDevRef 2"=w368:T3)  [unwired: 7 in]
          n137 = call <vilib>:"WPI_RobotDriveTankDrive.vi"("error in (no error)"=w367, "Right axis value"=0.0, "Left axis value"=0.0, "RobotDriveDevRef"=w368) -> ()  [unwired: 5 in, 3 out]
        }
        frame "LL", "RL" {
          n138 = call <vilib>:"WPI_RobotDriveTankDrive.vi"("error in (no error)"=w434, "Right axis value"=0.82 ("Y axis value"), "Left axis value"=0.8 ("X axis value"), "RobotDriveDevRef"=w433) -> ("error out"=w440:errorcluster, "RobotDriveDevRef"=w439:T3)  [unwired: 5 in, 1 out]
          n139 = call <vilib>:"WPI_RobotDriveDelayAndUpdateSafety.vi"("error in (no error)"=w440, "Delay (s)"=1.4, "RobotDriveDevRef"=w439) -> ("error out"=w448:errorcluster, "RobotDriveDevRef 2"=w447:T3)  [unwired: 7 in]
          n140 = call-poly <vilib>:"WPI_RobotDriveArcadeDrive.vi"("error in (no error)"=w448, "Y axis value"=0.0, "RobotDriveDevRef"=w447) -> ("error out"=w442:errorcluster, "RobotDriveDevRef"=w445:T3)  [unwired: 6 in, 1 out]
          n141 = call <vilib>:"WPI_MotorControlSetOutput.vi"("error in (no error)"=w442, "Output"=0.0, "MotorControlDevRef"=w432) -> ("error out"=w443:errorcluster)  [unwired: 6 in, 2 out]
          n142 = call <vilib>:"WPI_MotorControlSetOutput.vi"("error in (no error)"=w443, "Output"=0.0, "MotorControlDevRef"=w431) -> ("error out"=w441:errorcluster)  [unwired: 6 in, 2 out]
          n143 = call <vilib>:"WPI_RobotDriveDelayAndUpdateSafety.vi"("error in (no error)"=w441, "Delay (s)"=0.5, "RobotDriveDevRef"=w445) -> ()  [unwired: 7 in, 2 out]
        }
      }
    }
    frame "SF" {
    }
    frame "scale L" {
      n144 = case shown="\"LL\", \"RL\", Default" w458 {
        tunnel: w457 -> [w528 w542]
        tunnel: w456 -> [w508 w540]
        tunnel: w455 -> [w509 w541]
        tunnel: w454 -> [w505 _]
        tunnel: w453 -> [w504 _]
        tunnel: w452 -> [w503 _]
        tunnel: w451 -> [_ w543]
        tunnel: w450 -> [w472 _]
        frame "LL", "RL", Default {
          # "300in to scale"
          n145 = call <vilib>:"WPI_SwitchGetLimitValue.vi"("error in (no error)"=w505, "SwitchDevRef"=w504) -> ("Switch Pressed"=w506:bool)  [unwired: 7 in, 2 out]
          n146 = call <vilib>:"WPI_RobotDriveTankDrive.vi"("Right axis value"=0.82 ("Y axis value"), "Left axis value"=0.8 ("X axis value"), "RobotDriveDevRef"=w528) -> ("error out"=w534:errorcluster, "RobotDriveDevRef"=w533:T3)  [unwired: 6 in, 1 out]
          n147 = case shown="False" w506 {
            tunnel: [-0.65 ("Output") 0.0 ("Output")] -> w507
            frame False {
            }
            frame True {
            }
          }
          n148 = call <vilib>:"WPI_RobotDriveDelayAndUpdateSafety.vi"("error in (no error)"=w534, "Delay (s)"=3.5, "RobotDriveDevRef"=w533) -> ("error out"=w526:errorcluster, "RobotDriveDevRef 2"=w527:T3)  [unwired: 7 in]
          n149 = call <vilib>:"WPI_RobotDriveTankDrive.vi"("error in (no error)"=w526, "Right axis value"=0.0, "Left axis value"=0.0, "RobotDriveDevRef"=w527) -> ("error out"=w523:errorcluster, "RobotDriveDevRef"=w521:T3)  [unwired: 5 in, 1 out]
          n150 = call <vilib>:"WPI_MotorControlSetOutput.vi"("error in (no error)"=w523, "Output"=w507, "MotorControlDevRef"=w503) -> ("error out"=w520:errorcluster, "MotorControlDevRef"=w502:T4)  [unwired: 6 in, 1 out]
          n151 = call <vilib>:"WPI_RobotDriveDelayAndUpdateSafety.vi"("error in (no error)"=w520, "Delay (s)"=2.0, "RobotDriveDevRef"=w521) -> ("error out"=w514:errorcluster, "RobotDriveDevRef 2"=w515:T3)  [unwired: 7 in]
          n152 = call <vilib>:"WPI_RobotDriveTankDrive.vi"("error in (no error)"=w514, "Right axis value"=0.0, "Left axis value"=0.6, "RobotDriveDevRef"=w515) -> ("error out"=w501:errorcluster, "RobotDriveDevRef"=w516:T3)  [unwired: 5 in, 1 out]
          n153 = call <vilib>:"WPI_MotorControlSetOutput.vi"("error in (no error)"=w501, "Output"=0.0, "MotorControlDevRef"=w502) -> ("error out"=w475:errorcluster)  [unwired: 6 in, 2 out]
          n154 = call <vilib>:"WPI_RobotDriveDelayAndUpdateSafety.vi"("error in (no error)"=w475, "Delay (s)"=1.2, "RobotDriveDevRef"=w516) -> ("error out"=w510:errorcluster, "RobotDriveDevRef 2"=w511:T3)  [unwired: 7 in]
          n155 = call <vilib>:"WPI_RobotDriveTankDrive.vi"("error in (no error)"=w510, "Right axis value"=0.0, "Left axis value"=0.0, "RobotDriveDevRef"=w511) -> ("error out"=w474:errorcluster, "RobotDriveDevRef"=w486:T3)  [unwired: 5 in, 1 out]
          n156 = call <vilib>:"WPI_MotorControlSetOutput.vi"("error in (no error)"=w474, "Output"=0.1, "MotorControlDevRef"=w472) -> ("error out"=w473:errorcluster, "MotorControlDevRef"=w464:T4)  [unwired: 6 in, 1 out]
          n157 = call <vilib>:"WPI_RobotDriveDelayAndUpdateSafety.vi"("error in (no error)"=w473, "Delay (s)"=0.025, "RobotDriveDevRef"=w486) -> ("error out"=w465:errorcluster, "RobotDriveDevRef 2"=w466:T3)  [unwired: 7 in]
          n158 = call <vilib>:"WPI_RobotDriveTankDrive.vi"("error in (no error)"=w465, "Right axis value"=0.0, "Left axis value"=0.0, "RobotDriveDevRef"=w466) -> ("error out"=w462:errorcluster, "RobotDriveDevRef"=w469:T3)  [unwired: 5 in, 1 out]
          n159 = call <vilib>:"WPI_MotorControlSetOutput.vi"("error in (no error)"=w462, "Output"=0.0, "MotorControlDevRef"=w464) -> ("error out"=w461:errorcluster)  [unwired: 6 in, 2 out]
          n160 = call <vilib>:"WPI_RobotDriveDelayAndUpdateSafety.vi"("error in (no error)"=w461, "Delay (s)"=0.1, "RobotDriveDevRef"=w469) -> ("error out"=w459:errorcluster, "RobotDriveDevRef 2"=w460:T3)  [unwired: 7 in]
          n161 = call <vilib>:"WPI_RobotDriveTankDrive.vi"("error in (no error)"=w459, "Right axis value"=0.0, "Left axis value"=0.0, "RobotDriveDevRef"=w460) -> ("error out"=w485:errorcluster, "RobotDriveDevRef"=w484:T3)  [unwired: 5 in, 1 out]
          n162 = call <vilib>:"WPI_MotorControlSetOutput.vi"("error in (no error)"=w485, "Output"=1.0, "MotorControlDevRef"=w509) -> ("error out"=w536:errorcluster, "MotorControlDevRef"=w493:T4)  [unwired: 6 in, 1 out]
          n163 = call <vilib>:"WPI_MotorControlSetOutput.vi"("error in (no error)"=w536, "Output"=-1.0, "MotorControlDevRef"=w508) -> ("error out"=w535:errorcluster, "MotorControlDevRef"=w492:T4)  [unwired: 6 in, 1 out]
          n164 = call <vilib>:"WPI_RobotDriveDelayAndUpdateSafety.vi"("error in (no error)"=w535, "Delay (s)"=0.5, "RobotDriveDevRef"=w484) -> ("error out"=w496:errorcluster, "RobotDriveDevRef 2"=w497:T3)  [unwired: 7 in]
          n165 = call <vilib>:"WPI_RobotDriveTankDrive.vi"("error in (no error)"=w496, "Right axis value"=-0.5, "Left axis value"=-0.5, "RobotDriveDevRef"=w497) -> ("error out"=w494:errorcluster, "RobotDriveDevRef"=w481:T3)  [unwired: 5 in, 1 out]
          n166 = call <vilib>:"WPI_MotorControlSetOutput.vi"("error in (no error)"=w494, "Output"=0.0, "MotorControlDevRef"=w493) -> ("error out"=w495:errorcluster)  [unwired: 6 in, 2 out]
          n167 = call <vilib>:"WPI_MotorControlSetOutput.vi"("error in (no error)"=w495, "Output"=0.0, "MotorControlDevRef"=w492) -> ("error out"=w480:errorcluster)  [unwired: 6 in, 2 out]
          n168 = call <vilib>:"WPI_RobotDriveDelayAndUpdateSafety.vi"("error in (no error)"=w480, "Delay (s)"=1.5, "RobotDriveDevRef"=w481) -> ("error out"=w476:errorcluster, "RobotDriveDevRef 2"=w477:T3)  [unwired: 7 in]
          n169 = call <vilib>:"WPI_RobotDriveTankDrive.vi"("error in (no error)"=w476, "Right axis value"=0.0, "Left axis value"=0.0, "RobotDriveDevRef"=w477) -> ()  [unwired: 5 in, 3 out]
        }
        frame "LRL", "RRR" {
          n170 = call <vilib>:"WPI_RobotDriveTankDrive.vi"("error in (no error)"=w543, "Right axis value"=0.82 ("Y axis value"), "Left axis value"=0.8 ("X axis value"), "RobotDriveDevRef"=w542) -> ("error out"=w549:errorcluster, "RobotDriveDevRef"=w548:T3)  [unwired: 5 in, 1 out]
          n171 = call <vilib>:"WPI_RobotDriveDelayAndUpdateSafety.vi"("error in (no error)"=w549, "Delay (s)"=1.4, "RobotDriveDevRef"=w548) -> ("error out"=w557:errorcluster, "RobotDriveDevRef 2"=w556:T3)  [unwired: 7 in]
          n172 = call-poly <vilib>:"WPI_RobotDriveArcadeDrive.vi"("error in (no error)"=w557, "Y axis value"=0.0, "RobotDriveDevRef"=w556) -> ("error out"=w551:errorcluster, "RobotDriveDevRef"=w554:T3)  [unwired: 6 in, 1 out]
          n173 = call <vilib>:"WPI_MotorControlSetOutput.vi"("error in (no error)"=w551, "Output"=0.0, "MotorControlDevRef"=w541) -> ("error out"=w552:errorcluster)  [unwired: 6 in, 2 out]
          n174 = call <vilib>:"WPI_MotorControlSetOutput.vi"("error in (no error)"=w552, "Output"=0.0, "MotorControlDevRef"=w540) -> ("error out"=w550:errorcluster)  [unwired: 6 in, 2 out]
          n175 = call <vilib>:"WPI_RobotDriveDelayAndUpdateSafety.vi"("error in (no error)"=w550, "Delay (s)"=0.5, "RobotDriveDevRef"=w554) -> ()  [unwired: 7 in, 2 out]
        }
      }
    }
  }
